vi "概率函数（离散）.vi"() -> ()   [LabVIEW 2018]
uses:
  <vilib>/gmath/statdist.llb/Binomial PF.vi
  <vilib>/gmath/NI_Gmath.lvlib
panel:
  in  "p":dbl=0.02
  in  "n":i32=100
  in  "停止":bool
  out "prob(x)":dbl=0.36787944117144233
  in  "x":i32
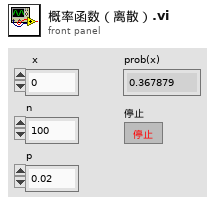
[diagram p1: front panel]
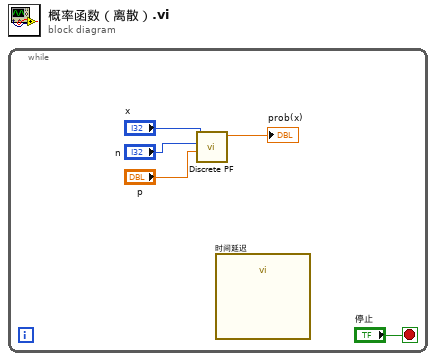
[diagram p0: block diagram]
diagram:
  n1 = while {
    stop <- "停止" stop-if-true
    n2 = call-poly <vilib>:"Discrete PF.vi"("p"="p", "n"="n", "x"="x") -> ("prob(x)"=→"prob(x)":dbl)  [unwired: 7 in, 1 out]
    n3 = call "时间延迟"() -> ()  [unwired: 11 in, 1 out]
  }
